vi "Write DC Motor Velocity Setpoints.vi"(8 "error in (no error)":errorcluster, 9 "right motor ccw velocity (rad/s)":dbl, 10 "left motor ccw velocity (rad/s)":dbl, 11 "starter kit host in":refnum<class "NI_Robotics_Starter Kit Host.lvclass">) -> (0 "error out":errorcluster, 3 "starter kit host out":refnum<class "NI_Robotics_Starter Kit Host.lvclass">)   [LabVIEW 2017, in "NI_Robotics_Starter Kit Host.lvclass"]
doc: "<B>Owning Palette:</B> Starter Kit 1.0 VIs, Starter Kit 2.0 VIs\n\nApplies velocity values to the drive motors on the Starter Kit robot. The left and right motors are defined by their positions as you view the robot from behind. The maximum motor velocity is 15.7 rad/s."
uses:
  <vilib>/robotics/Starter Kit/Host Interface/NI_Robotics_Starter Kit Host.lvclass
  <vilib>/robotics/Starter Kit/Host Interface/NI_Robotics_Starter Kit Host.lvclass/NI_Robotics_Starter Kit Host.ctl
  <instrlib>/DC Motor Controller/HAIOL/DC Motor Controller.lvclass
  <vilib>/robotics/Utilities/NI_Robotics Utilities.lvlib
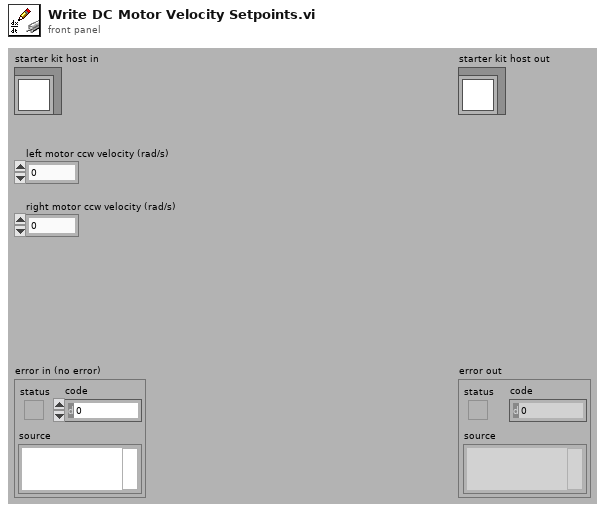
[diagram p1: front panel]
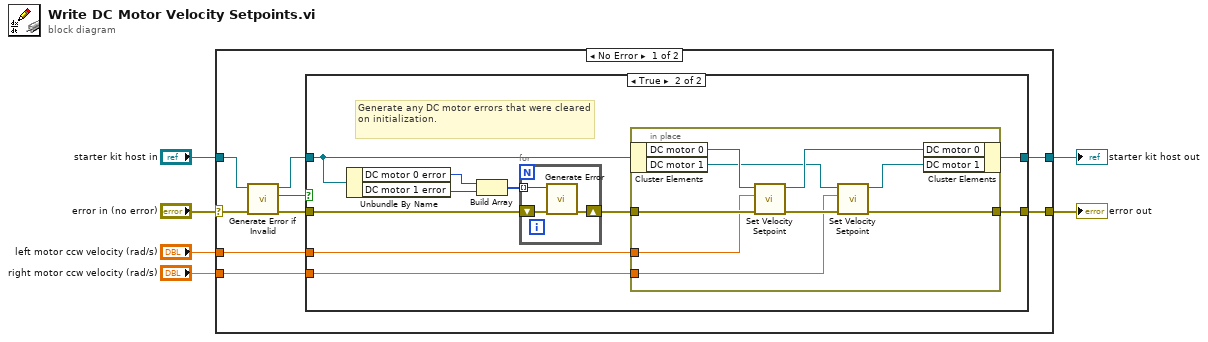
[diagram p0: block diagram]
diagram:
  n1 = case shown="No Error" "error in (no error)" {
    selector: "error in (no error)" -> [w11 w41]
    tunnel: [w14 w41] -> w5
    tunnel: [w15 w40] -> w3
    tunnel: "starter kit host in" -> [w9 w40]
    tunnel: "left motor ccw velocity (rad/s)" -> [w13 _]
    tunnel: "right motor ccw velocity (rad/s)" -> [w12 _]
    frame No Error {
      n2 = call <vilib>:"Generate Error if Invalid.vi"("error in (no error)"=w11, "starter kit host in"=w9) -> ("error out"=w10:errorcluster, "valid?"=w7:bool, "starter kit host out"=w8:refnum<class "NI_Robotics_Starter Kit Host.lvclass">)  [unwired: 7 in]
      n3 = case shown="True" w7 {
        tunnel: [w17 w27] -> w15
        tunnel: [w16 w26] -> w14
        tunnel: w13 -> [_ w25]
        tunnel: w12 -> [_ w24]
        tunnel: w10 -> [w16 w19]
        tunnel: w8 -> [w17 w23]
        frame False {
        }
        frame True {
          # "Generate any DC motor errors that were cleared on initialization."
          n4 = Unbundle By Name(w23) -> ("DC motor 0 error"=w21:i32, "DC motor 1 error"=w20:i32)
          n5 = Build Array(w21, w20) -> (w22:i32[])
          n6 = for {
            shift-right: [w29] -> w18
            shift-left: w19 -> [w30]
            tunnel: w22 -> [w28] mode=indexing
            n7 = call <vilib>:"Generate Error.vi"("error in (no error)"=w30, "code"=w28) -> ("error out"=w29:errorcluster)  [unwired: 9 in]
          }
          n8 = in-place {
            in-place-border: [w34] -> w26
            in-place-border: w18 -> [w33]
            in-place-border: w25 -> [w32]
            in-place-border: w24 -> [w31]
            n9 = in-place-cluster #1(w23) -> ("DC motor 0"=w39:refnum<class "DC Motor Controller.lvclass">, "DC motor 1"=w37:refnum<class "DC Motor Controller.lvclass">)
            n10 = call-dynamic "Set Velocity Setpoint.vi"("error in (no error)"=w33, "CCW Velocity (0 rad/s)"=w32, "DC Motor Controller in"=w39) -> ("error out"=w35:errorcluster, "DC Motor Controller out"=w38:refnum<class "DC Motor Controller.lvclass">)  [unwired: 7 in]
            n11 = call-dynamic "Set Velocity Setpoint.vi"("error in (no error)"=w35, "CCW Velocity (0 rad/s)"=w31, "DC Motor Controller in"=w37) -> ("error out"=w34:errorcluster, "DC Motor Controller out"=w36:refnum<class "DC Motor Controller.lvclass">)  [unwired: 7 in]
            n12 = in-place-cluster #1("DC motor 0"=w38, "DC motor 1"=w36) -> (w27:refnum<class "NI_Robotics_Starter Kit Host.lvclass">)
          }
        }
      }
    }
    frame Error {
    }
  }
  "error out" <- w5
  "starter kit host out" <- w3
